vi "HF MTOL turbidimeter.vi"(4 "State":i16=-1, 5 "Time":dbl format="%.2f", 6 "Sensor Values":dbl[](array[numeric]), 7 "Set Points":dbl[](array[numeric])=[1.0]) -> (0 "required data":T7={"Set Point names"=["data interval (s)", "device ID"], "required number of setpoints"=2, "required number of sensors"=0, "Sensor names"=[]}, 3 "output value":dbl)   [LabVIEW 2019]
uses:
  modbusrtu/MB status.ctl
  modbusrtu/ProCoDA MB Request.ctl
  modbusrtu/Read Write.ctl
  byte swap.ctl
  modbusrtu/MB ID-Address.ctl
  modbusrtu/SerialParameters.ctl
  modbusrtu/MB cmd buffer.ctl
panel:
  in  "MB ID-Address":T1={"Serial Parameter"={"Mode"=enum."RTU", "Address"=0, "Address bytes"=enum."1 byte"}, "Start register"=30001}
  in  "MB status":T3={"ProCoDA Request"={"# registers"=2, "Data to write"=[], "data interval (s)"=0.0, "command"=enum."Read", "PC update (s)"=0.0, "byte swap"=enum."no swap", "data type"=enum."float16"}, "MB response"=[0.0], "new cmd"=TRUE, "error"={"status"=FALSE, "code"=0, "source"=""}, "MB update(s)"=0.0} {"MB update(s)" format="%.2g"; "ProCoDA Request"."PC update (s)" format="%.2f"; "ProCoDA Request"."# registers" min=1}
  # "Enter the correct information for this control code in the required data structure below. Then make the current value default by right clicking on the border of the data structure. Select \"data operations\" and then select \"make current value default\". These values will be displayed by process controller."
  # "set the address bytes\nalways 1 so far and starting register\nas default values to configure device"
  # "set the byte swap,\nregister number,\nread/write cmd\nas default value to configure device"
  # "HF turbidimeters have none for parity as default.\nNeed to change to Even!"
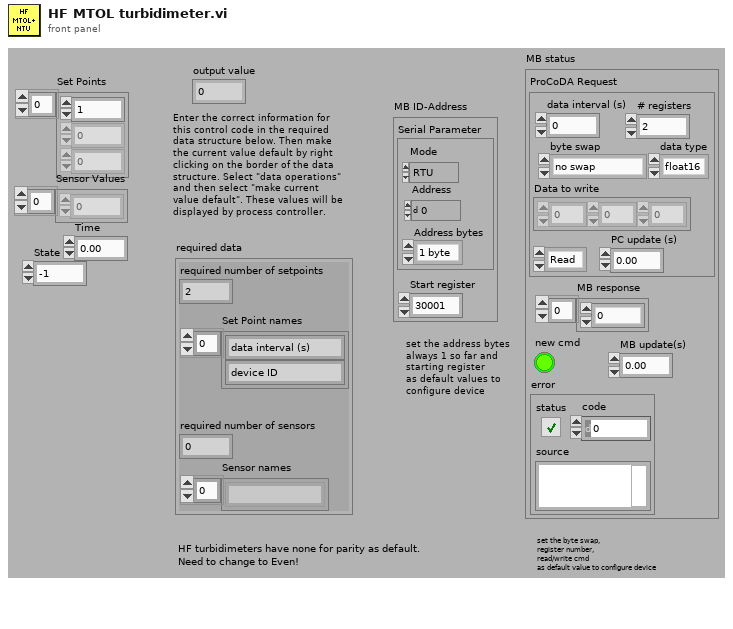
[diagram p1: front panel]
types:
  T1 = typedef "MB ID-Address.ctl" = cluster{"Serial Parameter":T2, "Start register":u16}
  T2 = typedef "SerialParameters.ctl" = cluster{"Mode":enum16{"RTU", "ASCII"}, "Address":u16, "Address bytes":enum16{"1 byte", "2 bytes"}}
  T3 = typedef "MB status.ctl" = cluster{"ProCoDA Request":T4, "MB response":dbl[], "new cmd":bool, "error":errorcluster, "MB update(s)":dbl}
  T4 = typedef "ProCoDA MB Request.ctl" = cluster{"# registers":u8, "Data to write":u16[], "data interval (s)":dbl, "command":T5, "PC update (s)":dbl, "byte swap":T6, "data type":enum16{"float16", "int16"}}
  T5 = typedef "Read Write.ctl" = enum16{"Read", "Write"}
  T6 = typedef "byte swap.ctl" = enum16{"no swap", "swap registers"}
  T7 = cluster{"Set Point names":string[], "required number of setpoints":u8, "required number of sensors":u8, "Sensor names":string[]}
  T8 = cluster{"Set Points[0]":dbl, "Set Points[1]":dbl}
  T9 = typedef "MB cmd buffer.ctl" = enum16{"ProCoDA", "MB succeed", "MB error", "MB Next Task", "ProCoDA read 1", "Commands pending"}
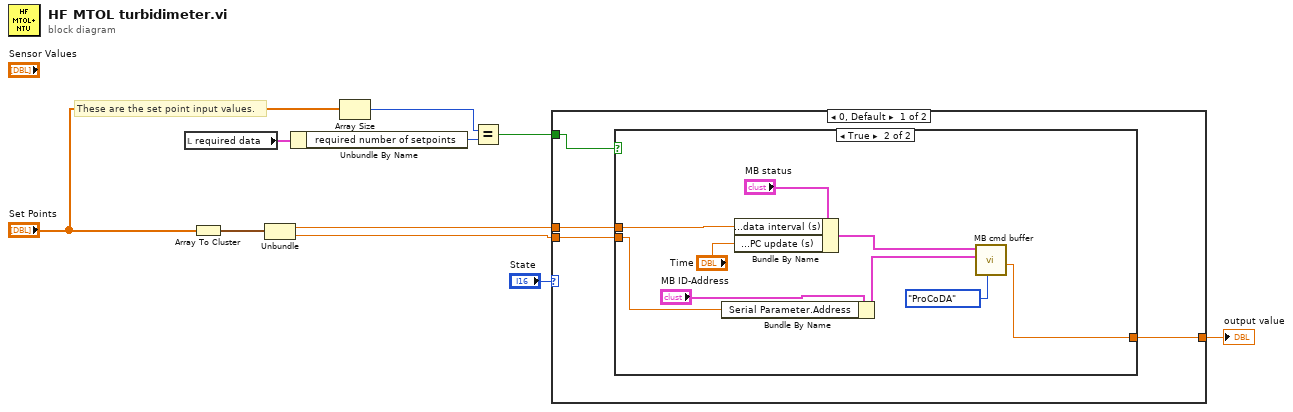
[diagram p0: block diagram]
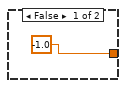
[diagram p2: hidden frame]
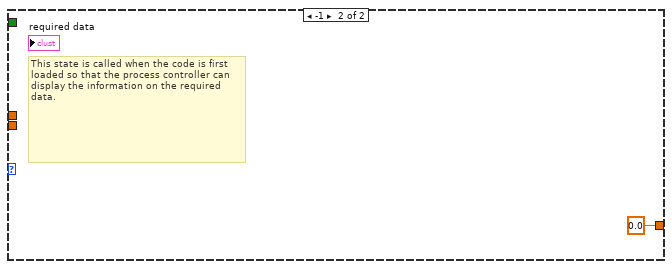
[diagram p3: hidden frame]
diagram:
  # "These are the set point input values."
  n1 = local read "required data"() -> (w6:T7)
  n2 = Array To Cluster(array="Set Points") -> (cluster=w3:T8)
  n3 = Unbundle(w3) -> ("Set Points[0]"=w2:dbl, "Set Points[1]"=w1:dbl)
  n4 = Unbundle By Name(w6) -> ("required number of setpoints"=w5:u8)
  n5 = Array Size(array="Set Points") -> (size(s)=w7:i32)
  n6 = Equal?(x=w7, y=w5) -> (x = y?=w4:bool)
  n7 = case shown="0, Default" "State" {
    tunnel: [w13 0.0 ("fraction on")] -> w9
    tunnel: w4 -> [w14 _]
    tunnel: w2 -> [w12 _]
    tunnel: w1 -> [w11 _]
    frame 0, Default {
      n8 = case shown="True" w14 {
        tunnel: [-1.0 ("fraction on") w18] -> w13
        tunnel: w12 -> [_ w21]
        tunnel: w11 -> [_ w19]
        frame False {
        }
        frame True {
          n9 = Bundle By Name(cluster="MB ID-Address", "Serial Parameter.Address"=w19) -> (w17:T1)
          n10 = Bundle By Name(cluster="MB status", "ProCoDA Request.data interval (s)"=w21, "ProCoDA Request.PC update (s)"="Time") -> (w22:T3)
          n11 = call "MB cmd buffer.vi"("MB cmd buffer"=MB_cmd_buffer."ProCoDA", "MB ID-Address in"=w17, "MB status in"=w22) -> ("output value"=w18:dbl)  [unwired: 2 in, 6 out]
        }
      }
    }
    frame -1 {
      # "This state is called when the code is first loaded so that the process controller can display the information on the required data."
    }
  }
  "output value" <- w9
